vi "Ini_GetBarcodeString.vi"(3 "error in (no error)":errorcluster, 5 "input cluster":T1={"Pinch-valve"="Test Sample", "XLP 6000 Pump"="MRJ", "Camera1"="", "Camera2"="", "Img_Capt"=FALSE, "Actuator"=FALSE, "Pump"=FALSE, "Cam 1"=FALSE, "Cam 2"=FALSE, "Empty_Refill"=FALSE, "Crop"=FALSE, "Light intensity"=0, "Exposure Time"=0.0, "Sample Name"="", "Operator"="", "Calibration 1"=path "C:/Users/au540322/Desktop/IHS_Project/images/Debris/Debris_0/Debris_0_2019_06_01-23-32-49-686.PNG", "Calibration 2"=path "C:/Users/au540322/Desktop/IHS_Project/images/Debris/Debris_0/Debris_0_2019_06_01-23-32-49-686.PNG", "Framerate"=100, "Timeout Sample"=500, "Collection date"="", "Sample size threshold"=500, "Empty start"=500, "Command"="", "Station"="", "Species Name"="", "Other Notes"="", "Aperture"=enum."Item 3", "Image Process Queue Size"=100, "Image Save Queue Size"=0, "Overload threshold"=0, "Max Framerate"=0, "Rectangle 1"={"Left"=0, "Top"=0, "Right"=0, "Bottom"=0, "Rotation"=0.0}, "Rectangle 2"={"Left"=0, "Top"=100, "Right"=100, "Bottom"=0, "Rotation"=0.0}, "Detection Region %"=200.0, "Detect 1"=path "C:/Users/au540322/Desktop/IHS_Project/images/Debris/Debris_0/Debris_0_2019_06_01-23-32-49-686.PNG", "Detect 2"=path "C:/Users/au540322/Desktop/IHS_Project/images/Debris/Debris_0/Debris_0_2019_06_01-23-32-49-686.PNG", "Max large object threshold"=500, "Open(T)/Close(F)"=FALSE, "Img_Capt Begin"=FALSE, "Dispense Speed"=0, "Flush Size"=0, "Location"="", "Latitude"="", "Longitude"="", "Determiner"="", "Sex"="", "Camera1_Img"=refnum, "Camera2_Img"=refnum, "Img1_Orig_Disp"=refnum, "Img2_Orig_Disp"=refnum, "Img1_Orig_RGB"=refnum, "Img2_Orig_RGB"=refnum, "Blue_Plane_Extract"=refnum, "Subtracted_Plane"=refnum, "Img1_Binary"=refnum, "Img2_Binary"=refnum, "Crop_Mask"=refnum, "Img1_Save"=refnum, "Img2_Save"=refnum, "Img1_Cali_Full"=refnum, "Img2_Cali_Full"=refnum, "Img1_Cali_Detect"=refnum, "Img2_Cali_Detect"=refnum, "Cam 1 queue"=refnum, "Cam 2 queue"=refnum, "Cam 1 - save queue"=refnum, "Cam 2 - save queue"=refnum, "Overlay_Ring"=0, "SystemVersion"=0, "System Serial"="", "Legacy Cam Attributes"=FALSE, "Camera Orientation 1"="", "Camera Orientation 2"="", "Pixel to mm 1"=0.0, "Pixel to mm 2"=0.0, "CAM1 Model"=enum."a2A5328-15ucBAS", "CAM2 Model"=enum."a2A5328-15ucBAS", "Flush Insect"=FALSE, "Pump Size"=FALSE, "Barcode"="", "Phase3"=FALSE, "Mega F3"="", "Container nr."=0.0, "Mannual F3"=TRUE} {"SystemVersion" items=["Standard", "XL"]; "Overlay_Ring" items=["Session Data", "Extended Setup", "Buffer", "Camera", "Dispenser", "Stats", "Connections"]; "Flush Size" min=1; "Dispense Speed" min=1; "Rectangle 2"."Rotation" format="%.2f"; "Rectangle 2"."Left" scale=0.0..1024.0; "Rectangle 2"."Right" scale=0.0..1024.0; "Rectangle 1"."Rotation" format="%.2f"; "Rectangle 1"."Left" scale=0.0..1024.0; "Rectangle 1"."Right" scale=0.0..1024.0; "Max Framerate" min=1; "Overload threshold" min=1; "Image Save Queue Size" min=1; "Image Process Queue Size" min=1; "Empty start" min=1; "Sample size threshold" min=1; "Framerate" min=1; "Light intensity" scale=0.0..100.0}) -> (0 "error out":errorcluster, 1 "F3 Status":string, 2 "Output Cluster":T1={"Pinch-valve"="Test Sample", "XLP 6000 Pump"="MRJ", "Camera1"="", "Camera2"="", "Img_Capt"=FALSE, "Actuator"=FALSE, "Pump"=FALSE, "Cam 1"=FALSE, "Cam 2"=FALSE, "Empty_Refill"=FALSE, "Crop"=FALSE, "Light intensity"=0, "Exposure Time"=0.0, "Sample Name"="", "Operator"="", "Calibration 1"=path "C:/Users/au540322/Desktop/IHS_Project/images/Debris/Debris_0/Debris_0_2019_06_01-23-32-49-686.PNG", "Calibration 2"=path "C:/Users/au540322/Desktop/IHS_Project/images/Debris/Debris_0/Debris_0_2019_06_01-23-32-49-686.PNG", "Framerate"=100, "Timeout Sample"=500, "Collection date"="", "Sample size threshold"=500, "Empty start"=500, "Command"="", "Station"="", "Species Name"="", "Other Notes"="", "Aperture"=enum."Item 3", "Image Process Queue Size"=100, "Image Save Queue Size"=0, "Overload threshold"=0, "Max Framerate"=0, "Rectangle 1"={"Left"=0, "Top"=0, "Right"=0, "Bottom"=0, "Rotation"=0.0}, "Rectangle 2"={"Left"=0, "Top"=100, "Right"=100, "Bottom"=0, "Rotation"=0.0}, "Detection Region %"=200.0, "Detect 1"=path "C:/Users/au540322/Desktop/IHS_Project/images/Debris/Debris_0/Debris_0_2019_06_01-23-32-49-686.PNG", "Detect 2"=path "C:/Users/au540322/Desktop/IHS_Project/images/Debris/Debris_0/Debris_0_2019_06_01-23-32-49-686.PNG", "Max large object threshold"=500, "Open(T)/Close(F)"=FALSE, "Img_Capt Begin"=FALSE, "Dispense Speed"=0, "Flush Size"=0, "Location"="", "Latitude"="", "Longitude"="", "Determiner"="", "Sex"="", "Camera1_Img"=refnum, "Camera2_Img"=refnum, "Img1_Orig_Disp"=refnum, "Img2_Orig_Disp"=refnum, "Img1_Orig_RGB"=refnum, "Img2_Orig_RGB"=refnum, "Blue_Plane_Extract"=refnum, "Subtracted_Plane"=refnum, "Img1_Binary"=refnum, "Img2_Binary"=refnum, "Crop_Mask"=refnum, "Img1_Save"=refnum, "Img2_Save"=refnum, "Img1_Cali_Full"=refnum, "Img2_Cali_Full"=refnum, "Img1_Cali_Detect"=refnum, "Img2_Cali_Detect"=refnum, "Cam 1 queue"=refnum, "Cam 2 queue"=refnum, "Cam 1 - save queue"=refnum, "Cam 2 - save queue"=refnum, "Overlay_Ring"=0, "SystemVersion"=0, "System Serial"="", "Legacy Cam Attributes"=FALSE, "Camera Orientation 1"="", "Camera Orientation 2"="", "Pixel to mm 1"=0.0, "Pixel to mm 2"=0.0, "CAM1 Model"=enum."a2A5328-15ucBAS", "CAM2 Model"=enum."a2A5328-15ucBAS", "Flush Insect"=FALSE, "Pump Size"=FALSE, "Barcode"="", "Phase3"=FALSE, "Mega F3"="", "Container nr."=0.0, "Mannual F3"=TRUE} {"SystemVersion" items=["Standard", "XL"]; "Overlay_Ring" items=["Session Data", "Extended Setup", "Buffer", "Camera", "Dispenser", "Stats", "Connections"]; "Flush Size" min=1; "Dispense Speed" min=1; "Rectangle 2"."Rotation" format="%.2f"; "Rectangle 2"."Left" scale=0.0..1024.0; "Rectangle 2"."Right" scale=0.0..1024.0; "Rectangle 1"."Rotation" format="%.2f"; "Rectangle 1"."Left" scale=0.0..1024.0; "Rectangle 1"."Right" scale=0.0..1024.0; "Max Framerate" min=1; "Overload threshold" min=1; "Image Save Queue Size" min=1; "Image Process Queue Size" min=1; "Empty start" min=1; "Sample size threshold" min=1; "Framerate" min=1; "Light intensity" scale=0.0..100.0})   [LabVIEW 2024]
uses:
  controls/Data.ctl
  <vilib>/userDefined/High Color/IMAQdx.ctl
  <vilib>/vision/Image Controls.llb/IMAQ Image.ctl
  ae539422-90c2-48c7-a089-5bb01302e7c9.vi
  d7fcdf58-1d6e-4c9b-b4c1-69249527c4a7.vi
  d9af6aa3-3436-4ca4-8cb3-b648403191fc.vi
  644cd9a0-6467-4848-a5d8-4a56f541d81a.vi
  179dc814-df1c-4c73-8a49-2a283ca76b51.vi
  612ec395-ea6c-4b3c-8db5-e19416acb38b.vi
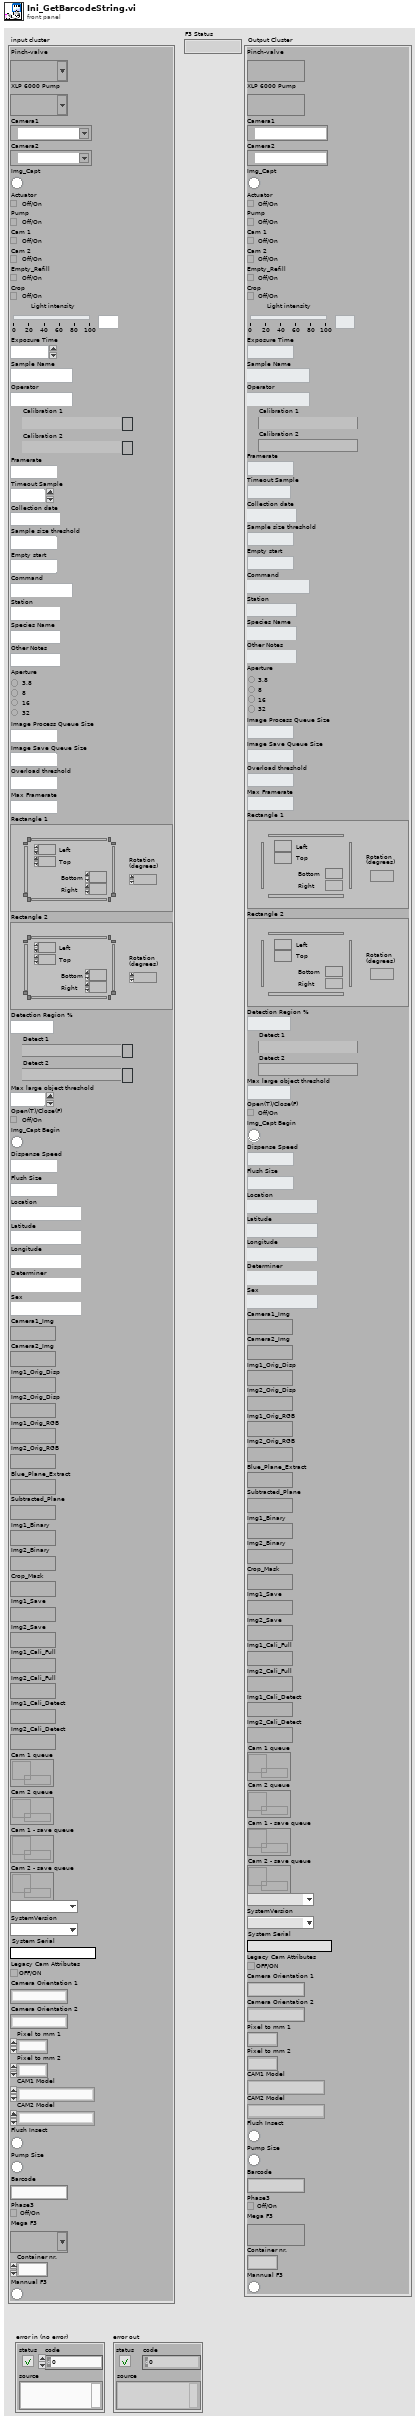
[diagram p1: front panel]
types:
  T1 = typedef "Data.ctl" = cluster{"Pinch-valve":refnum<visa-resource-name>, "XLP 6000 Pump":refnum<visa-resource-name>, "Camera1":T2, "Camera2":T2, "Img_Capt":bool, "Actuator":bool, "Pump":bool, "Cam 1":bool, "Cam 2":bool, "Empty_Refill":bool, "Crop":bool, "Light intensity":i32, "Exposure Time":dbl, "Sample Name":string, "Operator":string, "Calibration 1":path, "Calibration 2":path, "Framerate":i32, "Timeout Sample":i32, "Collection date":string, "Sample size threshold":i32, "Empty start":u32, "Command":string, "Station":string, "Species Name":string, "Other Notes":string, "Aperture":enum32{"Item 0", "Item 1", "Item 2", "Item 3"}, "Image Process Queue Size":i32, "Image Save Queue Size":i32, "Overload threshold":i32, "Max Framerate":i32, "Rectangle 1":T3, "Rectangle 2":T3, "Detection Region %":dbl, "Detect 1":path, "Detect 2":path, "Max large object threshold":i32, "Open(T)/Close(F)":bool, "Img_Capt Begin":bool, "Dispense Speed":i32, "Flush Size":i32, "Location":string, "Latitude":string, "Longitude":string, "Determiner":string, "Sex":string, "Camera1_Img":T4, "Camera2_Img":T4, "Img1_Orig_Disp":T4, "Img2_Orig_Disp":T4, "Img1_Orig_RGB":T4, "Img2_Orig_RGB":T4, "Blue_Plane_Extract":T4, "Subtracted_Plane":T4, "Img1_Binary":T4, "Img2_Binary":T4, "Crop_Mask":T4, "Img1_Save":T4, "Img2_Save":T4, "Img1_Cali_Full":T4, "Img2_Cali_Full":T4, "Img1_Cali_Detect":T4, "Img2_Cali_Detect":T4, "Cam 1 queue":refnum<queue>, "Cam 2 queue":refnum<queue>, "Cam 1 - save queue":refnum<queue>, "Cam 2 - save queue":refnum<queue>, "Overlay_Ring":u16, "SystemVersion":u16, "System Serial":string, "Legacy Cam Attributes":bool, "Camera Orientation 1":string, "Camera Orientation 2":string, "Pixel to mm 1":dbl, "Pixel to mm 2":dbl, "CAM1 Model":enum16{"a2A5328-15ucBAS", "acA1920-155uc"}, "CAM2 Model":enum16{"a2A5328-15ucBAS", "acA1920-155uc"}, "Flush Insect":bool, "Pump Size":bool, "Barcode":string, "Phase3":bool, "Mega F3":refnum<visa-resource-name>, "Container nr.":dbl, "Mannual F3":bool}
  T2 = typedef "IMAQdx.ctl" = refnum<k21>
  T3 = typedef "IMAQ Rectangle" = cluster{"Left":i32, "Top":i32, "Right":i32, "Bottom":i32, "Rotation":dbl}
  T4 = typedef "IMAQ Image.ctl" = refnum<image>
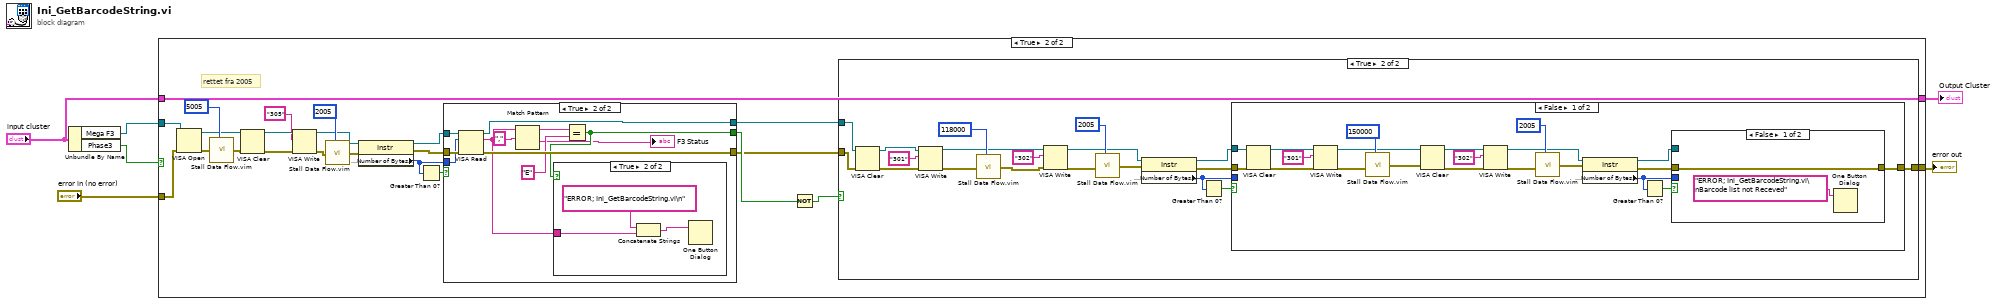
[diagram p0: block diagram]
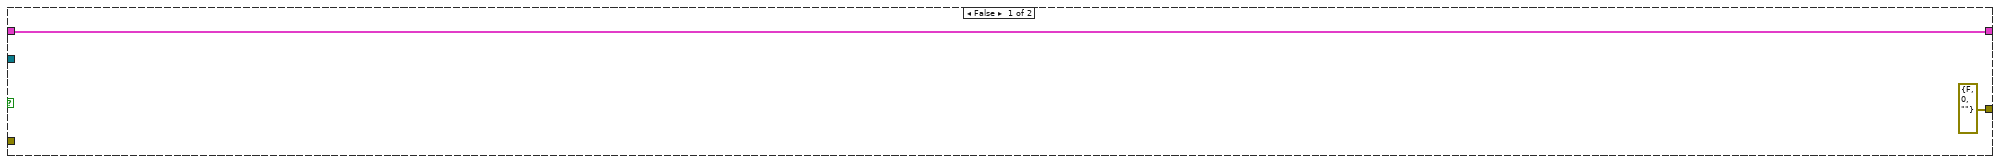
[diagram p2: hidden frame]
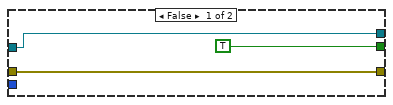
[diagram p3: hidden frame]
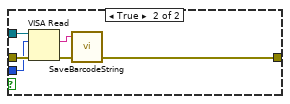
[diagram p6: hidden frame]
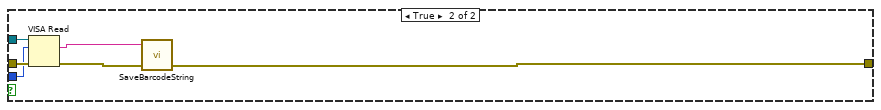
[diagram p7: hidden frame]
diagram:
  n1 = Unbundle By Name("input cluster") -> ("Mega F3"=w3:refnum<visa-resource-name>, "Phase3"=w4:bool)
  n2 = case shown="True" w4 {
    tunnel: "input cluster" -> [w8 w29]
    tunnel: [w8 w29] -> w5
    tunnel: [errorcluster {"status"=FALSE, "code"=0, "source"=""} ("error out") w31] -> w1
    tunnel: w3 -> [_ w20]
    tunnel: "error in (no error)" -> [_ w16]
    frame False {
    }
    frame True {
      # "rettet fra 2005"
      n3 = VISA Open(error in (no error)=w16, VISA resource name=w20) -> (VISA resource name=w12:refnum<visa-resource-name>, error out=w15:errorcluster)  [unwired: 3 in]
      n4 = call "Stall Data Flow.vim"("value in"=w15, "milliseconds to wait"=u32 5005) -> ("value out"=w14:errorcluster)  [unwired: 1 out]
      n5 = VISA Clear(VISA resource name=w12, error in (no error)=w14) -> (VISA resource name out=w28:refnum<visa-resource-name>, error out=w13:errorcluster)
      n6 = VISA Write(VISA resource name=w28, write buffer="305", error in (no error)=w13) -> (VISA resource name out=w9:refnum<visa-resource-name>, error out=w11:errorcluster)  [unwired: 1 out]
      n7 = call "Stall Data Flow.vim"("value in"=w11, "milliseconds to wait"=u32 2005) -> ("value out"=w10:errorcluster)  [unwired: 1 out]
      n8 = property class="Instr"(reference=w9, error in=w10) -> (reference out=w25:refnum<visa-resource-name>, error out=w24:errorcluster, "Serial Settings:Number of Bytes at Serial Port"=w26:u32)
      n9 = Greater Than 0?(x=w26) -> (x > 0?=w27:bool)
      n10 = case shown="True" w27 {
        tunnel: w26 -> [_ w43]
        tunnel: w25 -> [w34 w45]
        tunnel: w24 -> [w33 w44]
        tunnel: [w34 w42] -> w30
        tunnel: [w33 w41] -> w17
        tunnel: [TRUE w37] -> w18
        frame False {
        }
        frame True {
          n11 = VISA Read(VISA resource name=w45, byte count=w43, error in (no error)=w44) -> (VISA resource name out=w42:refnum<visa-resource-name>, read buffer=w36:string, error out=w41:errorcluster)  [unwired: 1 out]
          n12 = Match Pattern(string=w36, regular expression=",") -> (before substring=w38:string, after substring=→"F3 Status":string)  [unwired: 1 in, 2 out]
          n13 = Equal?(x=w38, y="E") -> (x = y?=w37:bool)
          n14 = case shown="True" w37 {
            tunnel: w36 -> [_ w46]
            frame False {
            }
            frame True {
              n15 = Concatenate Strings("ERROR; Ini_GetBarcodeString.vi\n", w46) -> (w47:string)
              n16 = One Button Dialog(message=w47) -> ()  [unwired: 1 in, 1 out]
            }
          }
        }
      }
      n17 = Not(x=w18) -> (.not. x?=w21:bool)
      n18 = case shown="True" w21 {
        tunnel: [w49 w61] -> w31
        tunnel: w30 -> [_ w59]
        tunnel: w17 -> [w49 w56]
        frame False {
        }
        frame True {
          n19 = VISA Clear(VISA resource name=w59, error in (no error)=w56) -> (VISA resource name out=w67:refnum<visa-resource-name>, error out=w65:errorcluster)
          n20 = VISA Write(VISA resource name=w67, write buffer="301", error in (no error)=w65) -> (VISA resource name out=w50:refnum<visa-resource-name>, error out=w52:errorcluster)  [unwired: 1 out]
          n21 = call "Stall Data Flow.vim"("value in"=w52, "milliseconds to wait"=u32 118000) -> ("value out"=w51:errorcluster)  [unwired: 1 out]
          n22 = VISA Write(VISA resource name=w50, write buffer="302", error in (no error)=w51) -> (VISA resource name out=w53:refnum<visa-resource-name>, error out=w55:errorcluster)  [unwired: 1 out]
          n23 = call "Stall Data Flow.vim"("value in"=w55, "milliseconds to wait"=u32 2005) -> ("value out"=w54:errorcluster)  [unwired: 1 out]
          n24 = property class="Instr"(reference=w53, error in=w54) -> (reference out=w63:refnum<visa-resource-name>, error out=w62:errorcluster, "Serial Settings:Number of Bytes at Serial Port"=w60:u32)
          n25 = Greater Than 0?(x=w60) -> (x > 0?=w64:bool)
          n26 = case shown="False" w64 {
            tunnel: w63 -> [w85 w103]
            tunnel: w62 -> [w84 w102]
            tunnel: [w83 w99] -> w61
            tunnel: w60 -> [_ w98]
            frame False {
              n27 = VISA Clear(VISA resource name=w85, error in (no error)=w84) -> (VISA resource name out=w87:refnum<visa-resource-name>, error out=w89:errorcluster)
              n28 = VISA Write(VISA resource name=w87, write buffer="301", error in (no error)=w89) -> (VISA resource name out=w72:refnum<visa-resource-name>, error out=w74:errorcluster)  [unwired: 1 out]
              n29 = call "Stall Data Flow.vim"("value in"=w74, "milliseconds to wait"=u32 150000) -> ("value out"=w73:errorcluster)  [unwired: 1 out]
              n30 = VISA Clear(VISA resource name=w72, error in (no error)=w73) -> (VISA resource name out=w77:refnum<visa-resource-name>, error out=w75:errorcluster)
              n31 = VISA Write(VISA resource name=w77, write buffer="302", error in (no error)=w75) -> (VISA resource name out=w69:refnum<visa-resource-name>, error out=w71:errorcluster)  [unwired: 1 out]
              n32 = call "Stall Data Flow.vim"("value in"=w71, "milliseconds to wait"=u32 2005) -> ("value out"=w70:errorcluster)  [unwired: 1 out]
              n33 = property class="Instr"(reference=w69, error in=w70) -> (reference out=w81:refnum<visa-resource-name>, error out=w80:errorcluster, "Serial Settings:Number of Bytes at Serial Port"=w79:u32)
              n34 = Greater Than 0?(x=w79) -> (x > 0?=w82:bool)
              n35 = case shown="False" w82 {
                tunnel: w81 -> [_ w97]
                tunnel: w80 -> [w91 w96]
                tunnel: [w91 w93] -> w83
                tunnel: w79 -> [_ w92]
                frame False {
                  n36 = One Button Dialog(message="ERROR; Ini_GetBarcodeString.vi\nBarcode list not Receved") -> ()  [unwired: 1 in, 1 out]
                }
                frame True {
                  n37 = VISA Read(VISA resource name=w97, byte count=w92, error in (no error)=w96) -> (read buffer=w94:string, error out=w95:errorcluster)  [unwired: 2 out]
                  n38 = call "SaveBarcodeString.vi"("error in"=w95, "String"=w94) -> ("error out"=w93:errorcluster)  [unwired: 3 in]
                }
              }
            }
            frame True {
              n39 = VISA Read(VISA resource name=w103, byte count=w98, error in (no error)=w102) -> (read buffer=w101:string, error out=w100:errorcluster)  [unwired: 2 out]
              n40 = call "SaveBarcodeString.vi"("error in"=w100, "String"=w101) -> ("error out"=w99:errorcluster)  [unwired: 3 in]
            }
          }
        }
      }
    }
  }
  "Output Cluster" <- w5
  "error out" <- w1
